vi "Y sensor convert meter to V.vi"() -> ()   [LabVIEW 2013]
doc: "This VI convert the displacement to voltage so that you will know what voltage you need to applied to Y peizo"
uses:
  Cypher XY LVDT Parameters.vi
panel:
  in  "Y coordinate":dbl format="%#_6p"
  out "Sensor Y Voltage":dbl
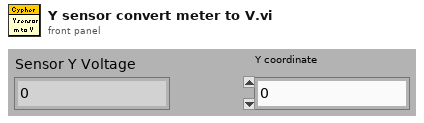
[diagram p1: front panel]
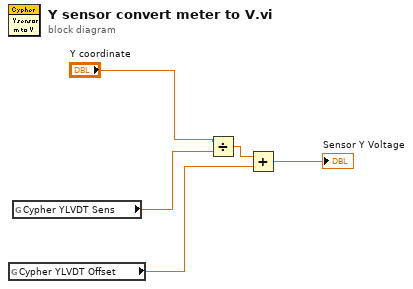
[diagram p0: block diagram]
diagram:
  n1 = global read "Cypher XY LVDT Parameters.vi" "Cypher YLVDT Offset"() -> (w2:dbl)
  n2 = global read "Cypher XY LVDT Parameters.vi" "Cypher YLVDT Sens"() -> (w4:dbl)
  n3 = Divide(x="Y coordinate", y=w4) -> (x/y=w3:dbl)
  n4 = Add(x=w3, y=w2) -> (x+y=→"Sensor Y Voltage":dbl)
